vi "pulses2commands.vi"(4 "N_pulses":i32=1 min=1, 6 "running_mode":enum16{"Continuous", "Single", "N pulses"}(ring), 8 "read_width_us":dbl=0.3, 9 "read_delay_us":dbl, 10 "pulse_width_us":dbl=50.0 format="%#.3f", 11 "pulse_period_us":dbl=100.0 format="%#_6p") -> (0 "error_out":errorcluster, 3 "instructions_array":T1(array[cluster]) {"Time" format="%#_6e"})   [LabVIEW 2018]
panel:
  # "Laser Pulse"
  # "Counting pulse"
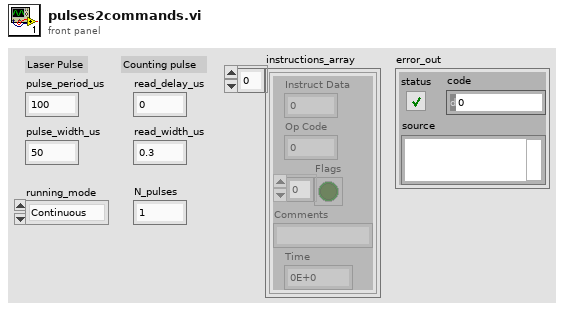
[diagram p1: front panel]
types:
  T1 = cluster{"Instruct Data":i32, "Op Code":i32, "Flags":bool[], "Comments":string, "Time":dbl}[]
  T2 = cluster{"Instruct Data":i32, "Op Code":i32, "Flags":bool[], "Comments":string, "Time":dbl}
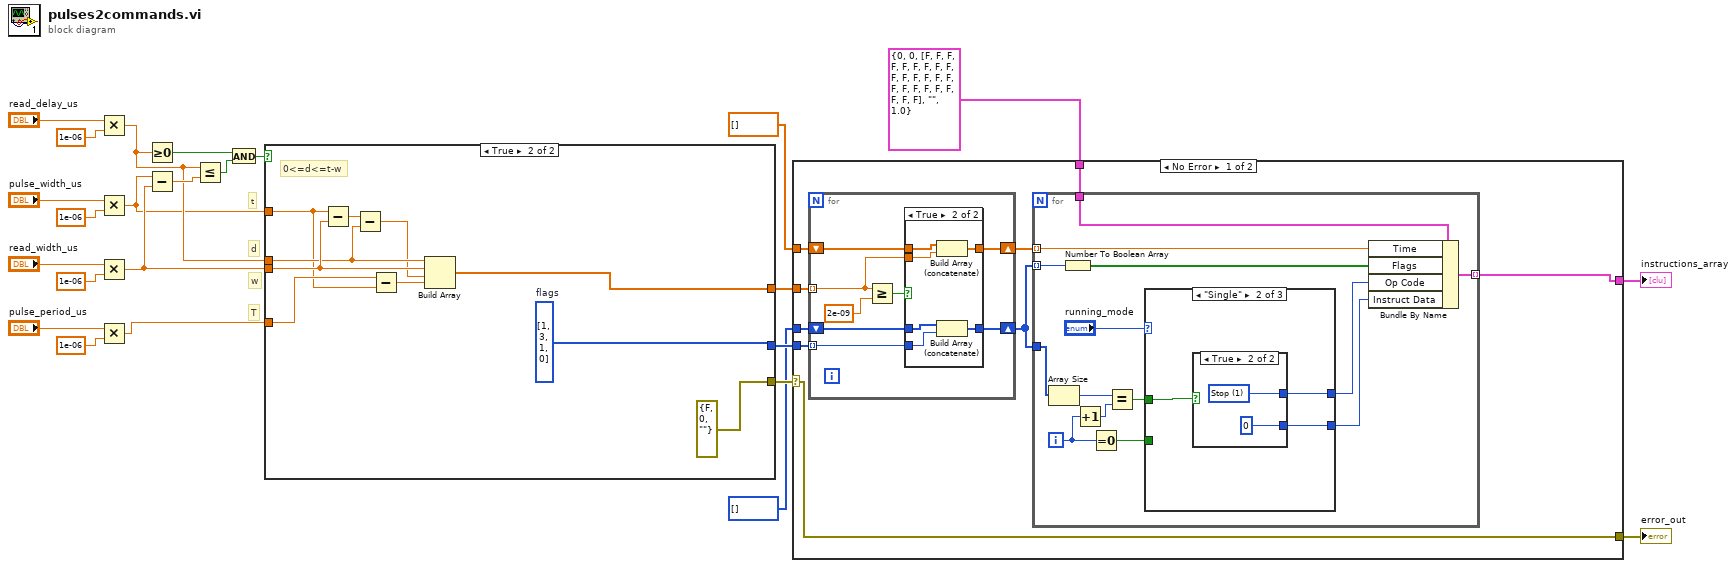
[diagram p0: block diagram]
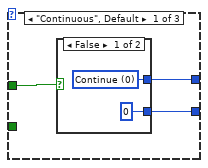
[diagram p2: hidden frame]
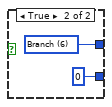
[diagram p3: hidden frame]
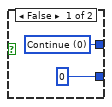
[diagram p4: hidden frame]
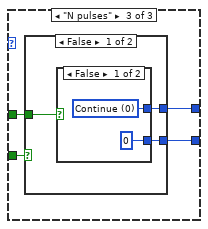
[diagram p5: hidden frame]
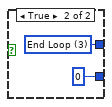
[diagram p6: hidden frame]
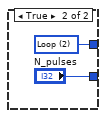
[diagram p7: hidden frame]
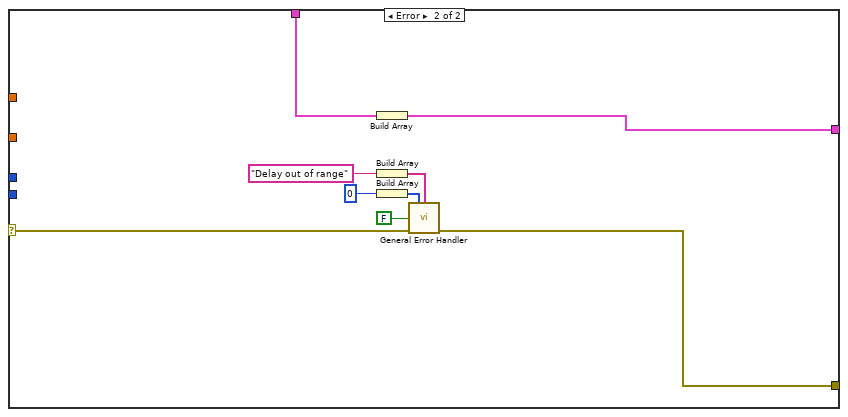
[diagram p9: hidden frame]
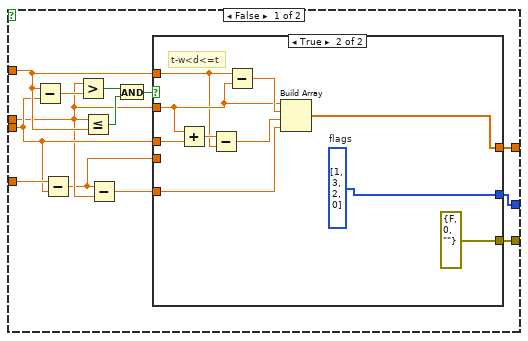
[diagram p10: hidden frame]
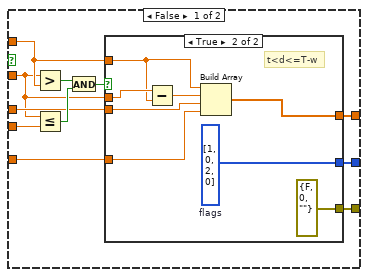
[diagram p11: hidden frame]
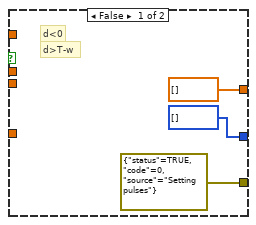
[diagram p12: hidden frame]
diagram:
  # "T"
  # "d"
  # "w"
  # "t"
  n1 = Multiply(x="read_delay_us", y=1e-06) -> (x*y=w12:dbl)
  n2 = Multiply(x="pulse_width_us", y=1e-06) -> (x*y=w4:dbl)
  n3 = Multiply(x="read_width_us", y=1e-06) -> (x*y=w16:dbl)
  n4 = Multiply(x="pulse_period_us", y=1e-06) -> (x*y=w1:dbl)
  n5 = Greater Or Equal To 0?(x=w12) -> (x >= 0?=w22:bool)
  n6 = Subtract(x=w4, y=w16) -> (x-y=w24:dbl)
  n7 = Less Or Equal?(x=w12, y=w24) -> (x <= y?=w23:bool)
  n8 = And(x=w22, y=w23) -> (x .and. y?=w21:bool)
  n9 = case shown="True" w21 {
    tunnel: w12 -> [w28 w77]
    tunnel: w16 -> [w29 w78]
    tunnel: w4 -> [w32 w71]
    tunnel: w1 -> [w33 w72]
    tunnel: [w30 w74] -> w19
    tunnel: [w26 w70] -> w20
    tunnel: [w25 errorcluster {"status"=FALSE, "code"=0, "source"=""} ("error constant")] -> w18
    frame False {
      n10 = Subtract(x=w32, y=w29) -> (x-y=w37:dbl)
      n11 = Subtract(x=w33, y=w29) -> (x-y=w27:dbl)
      n12 = Greater?(x=w28, y=w37) -> (0:w35:bool)
      n13 = Less Or Equal?(x=w28, y=w32) -> (x <= y?=w36:bool)
      n14 = Subtract(x=w27, y=w28) -> (x-y=w31:dbl)
      n15 = And(x=w35, y=w36) -> (x .and. y?=w34:bool)
      n16 = case shown="True" w34 {
        tunnel: w28 -> [w41 w68]
        tunnel: w32 -> [w44 w65]
        tunnel: w29 -> [w42 w67]
        tunnel: w31 -> [w43 w63]
        tunnel: [w40 w62] -> w30
        tunnel: w27 -> [w48 _]
        tunnel: [w39 w60] -> w26
        tunnel: [w38 errorcluster {"status"=FALSE, "code"=0, "source"=""} ("error constant")] -> w25
        frame False {
          n17 = Greater?(x=w41, y=w44) -> (0:w46:bool)
          n18 = Less Or Equal?(x=w41, y=w48) -> (x <= y?=w47:bool)
          n19 = And(x=w46, y=w47) -> (x .and. y?=w45:bool)
          n20 = case shown="True" w45 {
            tunnel: w44 -> [_ w55]
            tunnel: w43 -> [_ w59]
            tunnel: w42 -> [_ w58]
            tunnel: w41 -> [_ w56]
            tunnel: [dbl[] [] w54] -> w40
            tunnel: [u8[] [] ("flags") w52] -> w39
            tunnel: [errorcluster {"status"=TRUE, "code"=0, "source"="Setting pulses"} ("error constant") errorcluster {"status"=FALSE, "code"=0, "source"=""} ("error constant")] -> w38
            frame False {
              # "d>T-w"
              # "d<0"
            }
            frame True {
              w52 = u8[] [1, 0, 2, 0]  # flags
              # "t<d<=T-w"
              n21 = Subtract(x=w56, y=w55) -> (x-y=w57:dbl)
              n22 = Build Array(w55, w57, w58, w59) -> (w54:dbl[])
            }
          }
        }
        frame True {
          w60 = u8[] [1, 3, 2, 0]  # flags
          # "t-w<d<=t"
          n23 = Add(x=w68, y=w67) -> (x+y=w66:dbl)
          n24 = Subtract(x=w66, y=w65) -> (x-y=w64:dbl)
          n25 = Subtract(x=w65, y=w68) -> (x-y=w69:dbl)
          n26 = Build Array(w68, w69, w64, w63) -> (w62:dbl[])
        }
      }
    }
    frame True {
      w70 = u8[] [1, 3, 1, 0]  # flags
      # "0<=d<=t-w"
      n27 = Subtract(x=w71, y=w78) -> (x-y=w79:dbl)
      n28 = Subtract(x=w79, y=w77) -> (x-y=w76:dbl)
      n29 = Subtract(x=w72, y=w71) -> (x-y=w75:dbl)
      n30 = Build Array(w77, w78, w76, w75) -> (w74:dbl[])
    }
  }
  n31 = case shown="No Error" w18 {
    selector: w18 -> [w84 w152]
    tunnel: w20 -> [w82 _]
    tunnel: w19 -> [w86 _]
    tunnel: [w80 w154] -> w11
    tunnel: T2 {"Instruct Data"=0, "Op Code"=0, "Flags"=[FALSE, FALSE, FALSE, FALSE, FALSE, FALSE, FALSE, FALSE, FALSE, FALSE, FALSE, FALSE, FALSE, FALSE, FALSE, FALSE, FALSE, FALSE, FALSE, FALSE, FALSE, FALSE, FALSE, FALSE], "Comments"="", "Time"=1.0} ("PB Instruction") -> [w85 w153]
    tunnel: [w84 w151] -> w9
    tunnel: dbl[] [] ("appended array") -> [w83 _]
    tunnel: u8[] [] ("appended array") -> [w81 _]
    frame No Error {
      n32 = for {
        shift-right: [w134] -> w87
        shift-left: w81 -> [w136]
        shift-right: [w135] -> w88
        shift-left: w83 -> [w137]
        tunnel: w86 -> [w131] mode=indexing
        tunnel: w82 -> [w130] mode=indexing
        n33 = Greater Or Equal?(x=w131, y=2e-09) -> (x >= y?=w133:bool)
        n34 = case shown="True" w133 {
          tunnel: w137 -> [w138 w145]
          tunnel: w136 -> [w139 w141]
          tunnel: [w138 w144] -> w135
          tunnel: [w139 w142] -> w134
          tunnel: w131 -> [_ w143]
          tunnel: w130 -> [_ w140]
          frame False {
          }
          frame True {
            n35 = Build Array (concatenate)(w145, w143) -> (w144:dbl[])
            n36 = Build Array (concatenate)(w141, w140) -> (w142:u8[])
          }
        }
      }
      n37 = for {
        tunnel: w88 -> [w102] mode=indexing
        tunnel: w87 -> [w101] mode=indexing
        tunnel: [w95] -> w80 mode=indexing
        tunnel: w87 -> [w96]
        tunnel: w85 -> [w99]
        i -> [w93]
        n38 = Array Size(array=w96) -> (size(s)=w97:i32)
        n39 = Number To Boolean Array(number=w101) -> (Boolean array=w100:bool[])
        n40 = Increment(x=w93) -> (x+1=w98:i32)
        n41 = Equal To 0?(x=w93) -> (x = 0?=w91:bool)
        n42 = Equal?(x=w97, y=w98) -> (x = y?=w92:bool)
        n43 = case shown="\"Single\"" "running_mode" {
          tunnel: w92 -> [w103 w110 w120]
          tunnel: [w105 w112 w119] -> w90
          tunnel: [w104 w111 w118] -> w89
          tunnel: w91 -> [_ _ w117]
          frame "Continuous", Default {
            n44 = case shown="False" w103 {
              tunnel: [w107 w109] -> w105
              tunnel: [0 ("N_pulses") 0 ("N_pulses")] -> w104
              frame False {
                w107 = 0 items=["Continue", "Stop", "Loop", "End Loop", "JSR", "RTS", "Branch", "Long Delay", "Wait"] ("Op Code")
              }
              frame True {
                w109 = 6 items=["Continue", "Stop", "Loop", "End Loop", "JSR", "RTS", "Branch", "Long Delay", "Wait"] ("Op Code")
              }
            }
          }
          frame "Single" {
            n45 = case shown="True" w110 {
              tunnel: [w114 w116] -> w112
              tunnel: [0 ("N_pulses") 0 ("N_pulses")] -> w111
              frame False {
                w114 = 0 items=["Continue", "Stop", "Loop", "End Loop", "JSR", "RTS", "Branch", "Long Delay", "Wait"] ("Op Code")
              }
              frame True {
                w116 = 1 items=["Continue", "Stop", "Loop", "End Loop", "JSR", "RTS", "Branch", "Long Delay", "Wait"] ("Op Code")
              }
            }
          }
          frame "N pulses" {
            n46 = case shown="False" w117 {
              tunnel: w120 -> [w121 _]
              tunnel: [w123 w129] -> w119
              tunnel: [w122 "N_pulses"] -> w118
              frame False {
                n47 = case shown="False" w121 {
                  tunnel: [w125 w127] -> w123
                  tunnel: [0 ("N_pulses") 0 ("N_pulses")] -> w122
                  frame False {
                    w125 = 0 items=["Continue", "Stop", "Loop", "End Loop", "JSR", "RTS", "Branch", "Long Delay", "Wait"] ("Op Code")
                  }
                  frame True {
                    w127 = 3 items=["Continue", "Stop", "Loop", "End Loop", "JSR", "RTS", "Branch", "Long Delay", "Wait"] ("Op Code")
                  }
                }
              }
              frame True {
                w129 = 2 items=["Continue", "Stop", "Loop", "End Loop", "JSR", "RTS", "Branch", "Long Delay", "Wait"] ("Op Code")
              }
            }
          }
        }
        n48 = Bundle By Name(cluster=w99, "Time"=w102, "Flags"=w100, "Op Code"=w90, "Instruct Data"=w89) -> (w95:T2)
      }
    }
    frame Error {
      n49 = Build Array(w153) -> (w154:T1)
      n50 = Build Array("Delay out of range") -> (w148:string[])
      n51 = Build Array(0) -> (w146:i32[])
      n52 = call <vilib>:"General Error Handler.vi"("[user-defined codes]"=w146, "[user-defined descriptions]"=w148, "search ni.com link visible?(T)"=FALSE, "error in (no error)"=w152) -> ("error out"=w151:errorcluster)  [unwired: 7 in, 4 out]
    }
  }
  "instructions_array" <- w11
  "error_out" <- w9
